vi "Test Customer Pick Up Last Order Item Stops if in App Context.vi"(8 "error in (no error)":errorcluster, 11 "Customer Test in":refnum<class "Customer Test.lvclass">) -> (0 "error out":errorcluster, 3 "Customer Test out":refnum<class "Customer Test.lvclass">)   [LabVIEW 2020, in "Customer Test.lvclass"]
uses:
  Customer Test.lvclass
  C:/Program Files (x86)/National Instruments/LabVIEW 2020/vi.lib/Astemes/LUnit/Test Case.lvclass
  Processes/People/Customers/Customer/Customer.lvclass
  C:/Git/astemes-triarc-examples/Coffee Shop/Processes/People/Person/Person.lvclass
  C:/Program Files (x86)/National Instruments/LabVIEW 2020/vi.lib/Astemes/Triarc Framework/Process/Process.lvclass
  Support/Beverages/Beverage/Beverage.lvclass
  Support/Beverages/TypeDefs/Drink Type.ctl
  Support/Beverages/TypeDefs/Options.ctl
  <vilib>/Astemes/Triarc Framework/Process/Public/Lifecycle/Lifecycle State.ctl
  <vilib>/Astemes/Triarc Framework/Application/Application.lvclass
  Test Doubles/Stub Job Handler/Stub Job Handler.lvclass
  C:/Git/astemes-triarc-examples/Coffee Shop/Processes/People/Process Job/Job Handler.lvclass
  Processes/People/Person/Person.lvclass/Person.ctl
  <vilib>/Astemes/LUnit/Test Case.lvclass/Test Case.ctl
  <vilib>/Astemes/Triarc Framework/Process/Process.lvclass/Process.ctl
  <vilib>/Astemes/Triarc Framework/Application/Application.lvclass/Application.ctl
  <vilib>/Astemes/Triarc Framework/Application/Private/Add Process to Map.vi
  <vilib>/Astemes/Triarc Framework/Application/Private/Throw Error If Process Already in App.vi
  <vilib>/Astemes/Triarc Framework/Process/Protected/Messaging/Send Message.vi
  <vilib>/Astemes/Triarc Framework/Process/Public/Lifecycle/Get Lifecycle State.vi
  <vilib>/Astemes/Triarc Framework/Process/Protected/SubVIs/Set Context.vi
  <vilib>/Astemes/LUnit/Set Assertion Type.vi
  <vilib>/Astemes/LUnit/Palette/Pass.vi
  <vilib>/Astemes/LUnit/Palette/Fail.vi
  <vilib>/Astemes/Triarc Framework/Process/Private/SubVIs/Wait for finish.vi
  <vilib>/Astemes/Triarc Framework/Process/Private/SubVIs/Set Lifecycle State.vi
  <vilib>/Astemes/Triarc Framework/Application/Public/Get Process.vi
  <vilib>/Astemes/Triarc Framework/Process/Private/SubVIs/Handle Debug Data.vi
  <vilib>/Utility/error.llb/Clear Errors.vi
  <vilib>/Astemes/Triarc Framework/Process/Public/Lifecycle/Leave Process Loop.vi
  <vilib>/Astemes/LUnit/Add test result.vi
  <vilib>/Astemes/Triarc Framework/Application/Private/Retrieve Process from App.vi
  <vilib>/Astemes/Triarc Framework/Application/Private/Parse Process Name.vi
  <vilib>/Astemes/Triarc Framework/Application/Private/Get Process from Map.vi
  <vilib>/Astemes/Triarc Framework/Logging/Log Debug.vi
  <vilib>/AdvancedString/1D String Array to Delimited String.vi
  <vilib>/Utility/High Resolution Relative Seconds.vi
  <vilib>/Astemes/LUnit/LUnit Record Assertion Result.vi
  <vilib>/Astemes/Triarc Framework/Process/Protected/Messaging/Request Message.vi
  <vilib>/AdvancedString/Delimited String to 1D String Array.vi
  <vilib>/Astemes/LUnit/LUnit Aggregate Assertion Results.vi
  <vilib>/Astemes/Triarc Framework/Process/Private/SubVIs/Enqueue Request Message.vi
  <vilib>/Astemes/LUnit/Method Result/LUnit Merge Status.vi
  <vilib>/Astemes/LUnit/LUnit Concatenate result strings.vi
  <vilib>/Utility/error.llb/Error Cluster From Error Code.vi
  <vilib>/Astemes/Triarc Framework/Process/Public/Read Name.vi
  <vilib>/Astemes/Triarc Framework/Process/Private/SubVIs/Wait for Response Message.vi
  <vilib>/Astemes/Triarc Framework/Process/Process.lvclass
  <vilib>/Astemes/LUnit/Test Case.lvclass
  Processes/People/Person/Person.lvclass
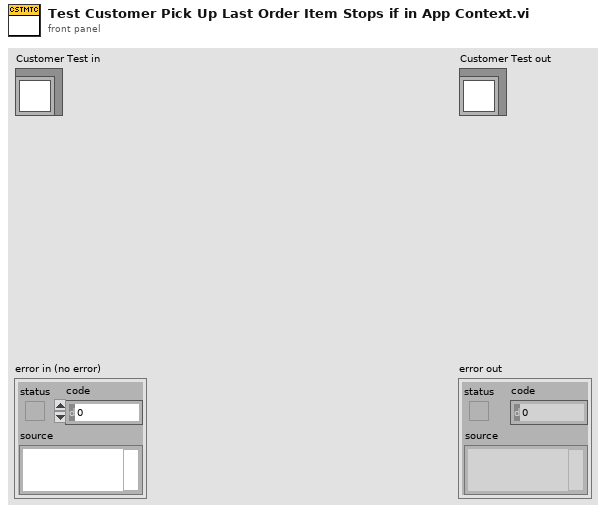
[diagram p1: front panel]
types:
  T1 = typedef "TF.lvlib/Process.lvclass/Lifecycle State.ctl" = enum16{"Uninitialized", "Initialized", "Started", "Running", "Stopped", "Finished"}
  T2 = typedef "Beverage.lvclass/Drink Type.ctl" = enum16{"Dark Roast", "Decaf", "Espresso", "House Blend"}
  T3 = typedef "Beverage.lvclass/Options.ctl" = enum16{"<None>", "Milk", "Mocha", "Soy", "Whip"}
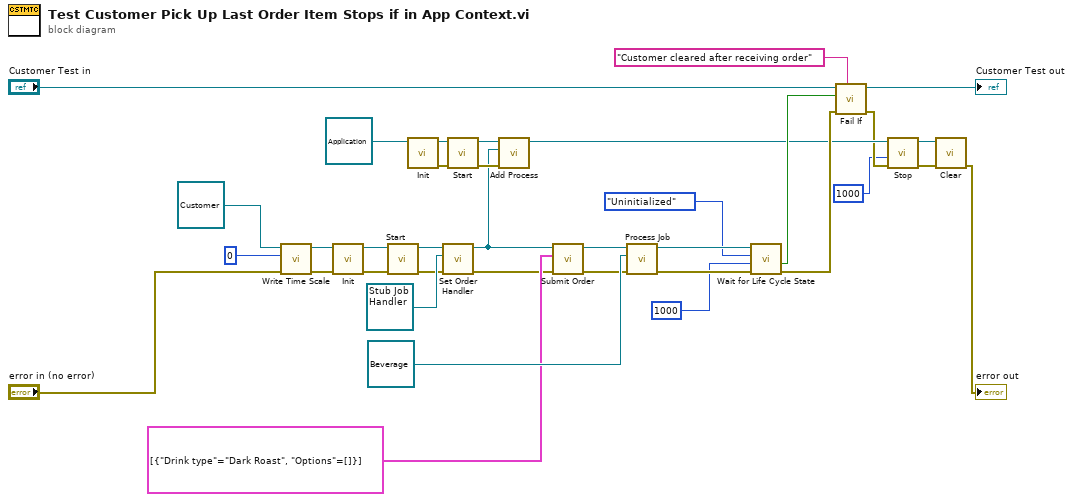
[diagram p0: block diagram]
diagram:
  n1 = call "Write Time Scale.vi"("error in (no error)"="error in (no error)", "Time Scale [ms]"=u32 0, "Person In"=refnum<class "Customer.lvclass"> refnum ("Customer.lvclass")) -> ("error out"=w7:errorcluster, "Person Out"=w5:refnum<class "Customer.lvclass">)  [unwired: 7 in]
  n2 = call-dynamic "Init.vi"("error in (no error)"=w7, "View In"=w5) -> ("error out"=w35:errorcluster, "View Out"=w2:refnum<class "Customer.lvclass">)  [unwired: 8 in]
  n3 = call <vilib>:"Start.vi"("error in (no error)"=w35, "Process In"=w2) -> ("error out"=w3:errorcluster, "Process Out"=w1:refnum<class "Customer.lvclass">)  [unwired: 7 in, 1 out]
  n4 = call-dynamic "Init.vi"("Process In"=refnum<class "Application.lvclass"> refnum ("TF.lvlib:Application.lvclass")) -> ("error out"=w20:errorcluster, "Process Out"=w21:refnum<class "Application.lvclass">)  [unwired: 9 in]
  n5 = call "Set Order Handler.vi"("error in (no error)"=w3, "Order Handler"=refnum<class "Stub Job Handler.lvclass"> refnum ("Stub Job Handler.lvclass"), "Customer In"=w1) -> ("error out"=w10:errorcluster, "Customer Out"=w9:refnum<class "Customer.lvclass">)  [unwired: 7 in]
  n6 = call <vilib>:"Start.vi"("error in (no error)"=w20, "Process In"=w21) -> ("error out"=w17:errorcluster, "Process Out"=w18:refnum<class "Application.lvclass">)  [unwired: 7 in, 1 out]
  n7 = call <vilib>:"Add Process.vi"("error in (no error)"=w17, "Process"=w9, "Application In"=w18) -> ("Application Out"=w16:refnum<class "Application.lvclass">)  [unwired: 7 in, 1 out]
  n8 = call "Submit Order.vi"("error in (no error)"=w10, "Order Content"=cluster{"Drink type":T2, "Options":T3[]}[] [{"Drink type"=enum."Dark Roast", "Options"=[]}], "Customer In"=w9) -> ("error out"=w27:errorcluster, "Customer Out"=w26:refnum<class "Customer.lvclass">)  [unwired: 7 in]
  n9 = call-dynamic "Process Job.vi"("error in (no error)"=w27, "Job"=refnum<class "Beverage.lvclass"> refnum ("Beverage.lvclass"), "Process Job In"=w26) -> ("error out"=w34:errorcluster, "Process Job Out"=w28:refnum<class "Customer.lvclass">)  [unwired: 7 in]
  n10 = call <vilib>:"Wait for Life Cycle State.vi"("error in (no error)"=w34, "timeout in ms (-1)"=1000, "Lifecycle State"=Lifecycle_State."Uninitialized", "Process In"=w28) -> ("error out"=w29:errorcluster, "timed out?"=w22:bool)  [unwired: 5 in, 1 out]
  n11 = call <vilib>:"Fail If.vi"("Description"="Customer cleared after receiving order", "error in (no error)"=w29, "Fail?"=w22, "LUnit Test Case In"="Customer Test in") -> ("error out"=w13:errorcluster, "LUnit Test Case Out"=→"Customer Test out":refnum<class "Customer Test.lvclass">)  [unwired: 6 in]
  n12 = call <vilib>:"Stop.vi"("error in (no error)"=w13, "timeout in ms (-1)"=1000, "Process In"=w16) -> ("error out"=w14:errorcluster, "Process Out"=w15:refnum<class "Application.lvclass">)  [unwired: 6 in, 1 out]
  n13 = call-dynamic "Clear.vi"("error in (no error)"=w14, "Application In"=w15) -> ("error out"=→"error out":errorcluster)  [unwired: 9 in]
